vi "GV_CursorView.vi"(6 "pict in":picture, 8 "error in (no error)":errorcluster, 10 "Pos":cluster{"x":i16, "y":i16}, 11 "Gviewer in":refnum<class "Gviewer.lvclass">) -> (0 "error out":errorcluster, 3 "Gviewer out":refnum<class "Gviewer.lvclass">, 4 "pict out":picture)   [LabVIEW 2020, in "Sgraph_lib_V1.lvlib" / "Gviewer.lvclass"]
doc: "Andre Koelewijn, 11 aug 2021\n\nDraw cursor on canvas"
uses:
  Gviewer.lvclass
  Gviewer.lvclass/Gviewer.ctl
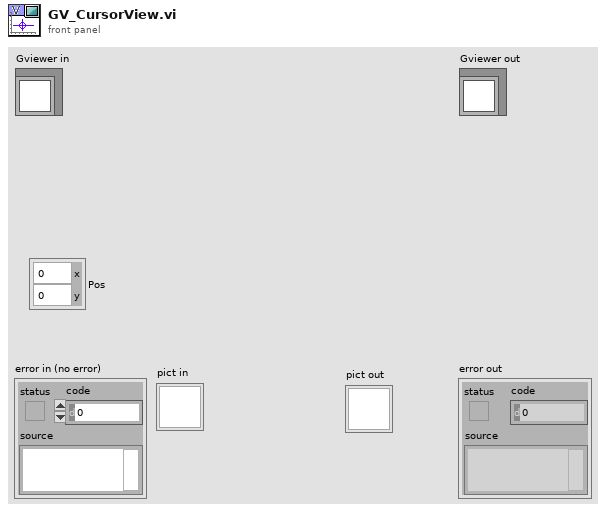
[diagram p1: front panel]
types:
  T1 = cluster{"Width":u16, "Style":enum32{"Solid", "Dash", "Dot", "DashDot", "DashDotDot"}}
  T2 = cluster{"horizontal":enum16{"left", "center", "right"}, "vertical":enum16{"top", "center", "bottom"}}
  T3 = typedef "Sgraph_lib_V1.lvlib/Gviewer.lvclass/Typedef_SelProperties.ctl" = cluster{"Color":u32, "LineType":T4, "max":dbl, "min":dbl, "unit":string}
  T4 = typedef "Sgraph_lib_V1.lvlib/Gviewer.lvclass/Typedef_LineType.ctl" = enum16{"num_bare", "num_MinMax_Area", "num_MinMax_Lines", "num_MinMax_Forfor", "num_Max_Area", "num_Max_Line", "num_Max_Forfor", "num_Min_Area", "num_Min_Line", "num_Min_Fosfor", "Boolean_Line_01", "Boolean_Area_01", "Boolean_Fosfor_01", "Boolean_Line_TF", "Boolean_Area_TF", "Boolean_Fosfor_TF", "Boolean_OnOff_Line", "Boolean_OnOff_Area", "Boolean_OnOff_Fosfor", "Boolean_spare", "StringEvent_Line", "StringEvent_TimeLine"}
  T5 = typedef "Sgraph_lib_V1.lvlib/DBAL.lvclass/DBAL_TAGprops.ctl" = T6[]
  T6 = typedef "Sgraph_lib_V1.lvlib/DBAL.lvclass/DBAL_TAGpropEdit.ctl" = cluster{"TAG":string, "Qtype":string, "TAGprop":T7}
  T7 = typedef "Sgraph_lib_V1.lvlib/typedef_com_TagProp.ctl" = cluster{"Description":string, "EngUnits":string, "RangeH":dbl, "RangeL":dbl, "Resolution":i32, "Obsolete":bool, "ChangeDate":timestamp, "ChangeSource":string, "ChangeReason":string, "TagFunc":u32}
  T8 = cluster{"data":dbl[], "max":dbl[], "min":dbl[], "Status":u32[]}[]
  T9 = cluster{"data":dbl[], "max":dbl[], "min":dbl[], "Status":u32[]}
  T10 = typedef "LVPositionTypeDef.ctl" = cluster{"Left":i32, "Top":i32}
  T11 = cluster{"left":i16, "top":i16, "right":i16, "bottom":i16}
  T12 = typedef "LVPoint32TypeDef.ctl" = cluster{"Horizontal":i32, "Vertical":i32}
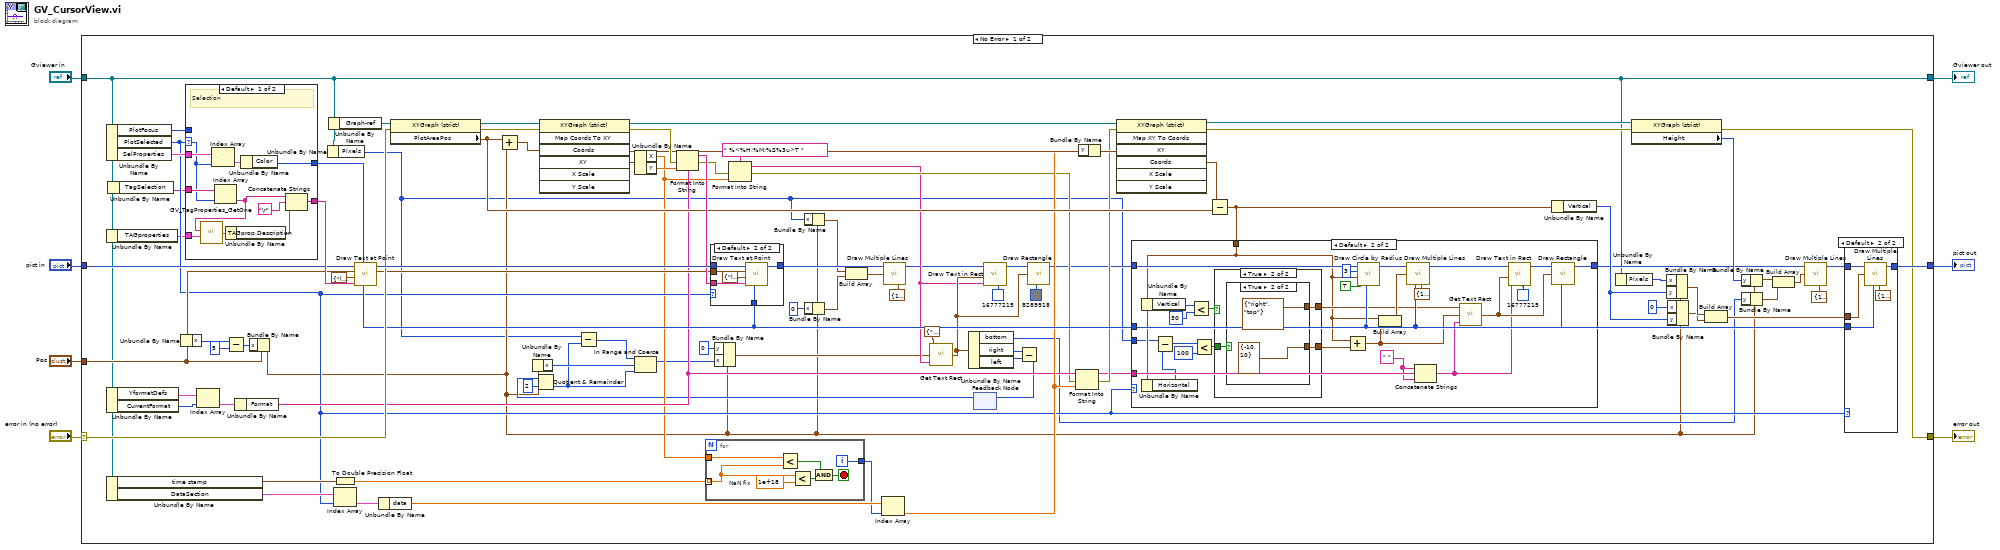
[diagram p0: block diagram]
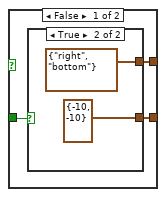
[diagram p3: hidden frame]
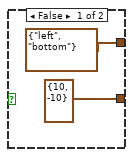
[diagram p4: hidden frame]
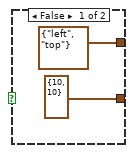
[diagram p5: hidden frame]
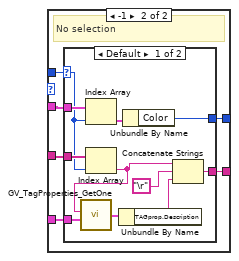
[diagram p8: hidden frame]
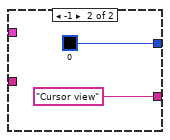
[diagram p9: hidden frame]
diagram:
  n1 = case shown="No Error" "error in (no error)" {
    selector: "error in (no error)" -> [w86 w193]
    tunnel: [w46 w193] -> w6
    tunnel: [w9 w192] -> w4
    tunnel: "Gviewer in" -> [w9 w192]
    tunnel: "pict in" -> [w89 w191]
    tunnel: [w49 w191] -> w2
    tunnel: "Pos" -> [w62 _]
    frame No Error {
      n2 = Unbundle By Name(w9) -> ("PlotFocus"=w52:i32, "PlotSelected"=w53:i32, "SelProperties"=w98:T3[])
      n3 = Unbundle By Name(w9) -> ("TAGproperties"=w8:T5)
      n4 = Unbundle By Name(w9) -> ("YformatDefs"=w81:cluster{"Description":string, "Format":string}[], "CurrentFormat"=w80:i32)
      n5 = Unbundle By Name(w9) -> ("time stamp"=w75:timestamp[], "DataSection"=w77:T8)
      n6 = Unbundle By Name(w9) -> ("TagSelection"=w10:string[])
      n7 = Unbundle By Name(w62) -> ("x"=w95:i16)
      n8 = case shown="Default" w53 {
        selector: w53 -> [w165 _]
        tunnel: w10 -> [w166 w174]
        tunnel: [w164 w177] -> w97
        tunnel: w98 -> [w169 w173]
        tunnel: [w170 w176] -> w59
        tunnel: w52 -> [_ w175]
        tunnel: w8 -> [w163 w172]
        frame Default {
          # "Selection"
          n9 = Index Array(array=w169, index=w165) -> (element=w171:T3)
          n10 = Index Array(array=w166, index=w165) -> (element=w162:string)
          n11 = call "GV_TagProperties_GetOne.vi"("TAG"=w162, "TAGproperties"=w163) -> ("TAGproperty"=w161:T6)  [unwired: 5 in]
          n12 = Unbundle By Name(w161) -> ("TAGprop.Description"=w168:string)
          n13 = Unbundle By Name(w171) -> ("Color"=w170:u32)
          n14 = Concatenate Strings(w162, "\r", w168) -> (w164:string)
        }
        frame -1 {
          # "No selection"
          n15 = case shown="Default" w175 {
            selector: w175 -> [w184 _]
            tunnel: [w181 "Cursor view"] -> w177
            tunnel: [w185 u32 0 ("Color")] -> w176
            tunnel: w174 -> [w188 _]
            tunnel: w173 -> [w187 _]
            tunnel: w172 -> [w180 _]
            frame Default {
              n16 = Index Array(array=w187, index=w184) -> (element=w186:T3)
              n17 = Index Array(array=w188, index=w184) -> (element=w179:string)
              n18 = call "GV_TagProperties_GetOne.vi"("TAG"=w179, "TAGproperties"=w180) -> ("TAGproperty"=w178:T6)  [unwired: 5 in]
              n19 = Unbundle By Name(w178) -> ("TAGprop.Description"=w183:string)
              n20 = Unbundle By Name(w186) -> ("Color"=w185:u32)
              n21 = Concatenate Strings(w179, "\r", w183) -> (w181:string)
            }
            frame -1 {
            }
          }
        }
      }
      n22 = Index Array(array=w81, index=w80) -> (element=w79:cluster{"Description":string, "Format":string})
      n23 = Subtract(x=w95, y=i16 5) -> (x-y=w93:i16)
      n24 = Unbundle By Name(w79) -> ("Format"=w57:string)
      n25 = Bundle By Name(cluster=w62, "x"=w93) -> (w16:cluster{"x":i16, "y":i16})
      n26 = Unbundle By Name(w9) -> ("Pixels"=w11:i32)
      n27 = Unbundle By Name(w9) -> ("Graph-ref"=w88:refnum<vi>)
      n28 = To Double Precision Float(number=w75) -> (double precision float=w74:dbl[])
      n29 = Index Array(array=w77, index=w53) -> (element=w76:T9)
      n30 = call <vilib>:"Draw Text at Point.vi"("text color(black)"=w59, "text"=w97, "alignment(left, top)"=T2 {"horizontal"=enum."left", "vertical"=enum."top"}, "origin"=w62, "picture"=w89) -> ("new picture"=w92:picture)  [unwired: 5 in, 1 out]
      n31 = Unbundle By Name(w76) -> ("data"=w73:dbl[])
      n32 = property class="XYGraph (strict)"(reference=w88, error in=w86) -> (reference out=w84:refnum<vi>, error out=w85:errorcluster, "PlotAreaPos"=w60:T10)
      n33 = Add(x=w60, y=w16) -> (x+y=w87:T10)
      n34 = Unbundle By Name(w16) -> ("x"=w35:i16)
      n35 = invoke class="XYGraph (strict)" method="Map Coords To XY"(reference=w84, error in=w85, "Coords"=w87) -> (reference out=w71:refnum<vi>, error out=w78:errorcluster, "XY"=w69:cluster{"X":dbl, "Y":dbl})  [unwired: 4 in, 4 out]
      n36 = Unbundle By Name(w69) -> ("X"=w50:dbl, "Y"=w83:dbl)
      n37 = Format Into String(format string=w57, error in=w78, w83) -> (resulting string=w82:string, error out=w48:errorcluster)  [unwired: 1 in]
      n38 = for {
        tunnel: w74 -> [w151] mode=indexing
        tunnel: w50 -> [w153]
        tunnel: [w152] -> w72
        i -> [w152]
        stop <- w147 stop-if-true
        w150 = 1e+18  # NaN fix
        n39 = Less?(x=w153, y=w151) -> (x < y?=w148:bool)
        n40 = Less?(x=w151, y=w150) -> (x < y?=w149:bool)
        n41 = And(x=w148, y=w149) -> (x .and. y?=w147:bool)
      }
      n42 = case shown="Default" w53 {
        tunnel: w92 -> [w154 w159]
        tunnel: [w154 w158] -> w25
        tunnel: w62 -> [_ w155]
        tunnel: w82 -> [_ w157]
        tunnel: w59 -> [_ w156]
        frame -1 {
        }
        frame Default {
          n43 = call <vilib>:"Draw Text at Point.vi"("text color(black)"=w156, "text"=w157, "alignment(left, top)"=T2 {"horizontal"=enum."left", "vertical"=enum."bottom"}, "origin"=w155, "picture"=w159) -> ("new picture"=w158:picture)  [unwired: 5 in, 1 out]
        }
      }
      n44 = Format Into String(format string=" %<%H:%M:%S%3u>T ", error in=w48, w50) -> (resulting string=w38:string, error out=w47:errorcluster)  [unwired: 1 in]
      n45 = Bundle By Name(cluster=w16, "x"=w11) -> (w21:cluster{"x":i16, "y":i16})
      n46 = Bundle By Name(cluster=w16, "x"=i16 0) -> (w22:cluster{"x":i16, "y":i16})
      n47 = Build Array(w21, w22) -> (w20:cluster{"x":i16, "y":i16}[])
      n48 = Index Array(array=w73, index=w72) -> (element=w58:dbl)
      n49 = call <vilib>:"Draw Multiple Lines.vi"("picture"=w25, "line endpoints"=w20, "pen"=T1 {"Width"=1, "Style"=enum."Dot"}) -> ("new picture"=w24:picture)  [unwired: 6 in]
      n50 = feedback #1() -> (w28:i16)  [unwired: 1 in]
      n51 = Quotient & Remainder(x=w28, y=i16 2) -> (floor(x/y)=w32:i16)  [unwired: 1 out]
      n52 = Subtract(x=w11, y=w32) -> (x-y=w33:i32)
      n53 = In Range and Coerce(upper limit=w33, x=w35, lower limit=w32) -> (coerced(x)=w34:i32)  [unwired: 1 out]
      n54 = Bundle By Name(cluster=w16, "y"=i16 0, "x"=w34) -> (w30:cluster{"x":i16, "y":i16})
      n55 = call <vilib>:"Get Text Rect.vi"("alignment(left, top)"=T2 {"horizontal"=enum."center", "vertical"=enum."top"}, "origin(0,0)"=w30, "text"=w38) -> ("rect"=w44:T11)  [unwired: 6 in]
      n56 = Unbundle By Name(w44) -> ("bottom"=w17:i16, "right"=w43:i16, "left"=w42:i16)
      n57 = call <vilib>:"Draw Text in Rect.vi"("BG color(transparent)"=u32 16777215, "text"=w38, "rect"=w44, "picture"=w24) -> ("new picture"=w45:picture)  [unwired: 7 in]
      n58 = Subtract(x=w43, y=w42) -> (x-y=w36:i16)
      n59 = feedback-in #1(w36) -> ()
      n60 = call <vilib>:"Draw Rectangle.vi"("picture"=w45, "rect"=w44, "color(black)"=u32 8289918 ("BG color(transparent)")) -> ("new picture"=w39:picture)  [unwired: 6 in]
      n61 = Format Into String(format string=w57, error in=w47, w58) -> (resulting string=w55:string, error out=w56:errorcluster)  [unwired: 1 in]
      n62 = Bundle By Name(cluster=w69, "Y"=w58) -> (w68:cluster{"X":dbl, "Y":dbl})
      n63 = invoke class="XYGraph (strict)" method="Map XY To Coords"(reference=w71, error in=w56, "XY"=w68) -> (reference out=w26:refnum<vi>, error out=w70:errorcluster, "Coords"=w63:T12)  [unwired: 4 in, 4 out]
      n64 = Subtract(x=w63, y=w60) -> (x-y=w54:T12)
      n65 = case shown="Default" w53 {
        tunnel: w39 -> [w99 w123]
        tunnel: [w99 w117] -> w18
        tunnel: w59 -> [_ w115]
        tunnel: w55 -> [_ w112]
        tunnel: w54 -> [_ w105]
        tunnel: w11 -> [_ w104]
        frame -1 {
        }
        frame Default {
          w110 = " "
          n66 = Unbundle By Name(w105) -> ("Vertical"=w109:i32)
          n67 = Unbundle By Name(w105) -> ("Horizontal"=w103:i32)
          n68 = Subtract(x=w104, y=w103) -> (x-y=w102:i32)
          n69 = Less?(x=w109, y=30) -> (x < y?=w107:bool)
          n70 = Less?(x=w102, y=100) -> (x < y?=w100:bool)
          n71 = case shown="True" w107 {
            tunnel: [w128 w135] -> w125
            tunnel: [w129 w136] -> w106
            tunnel: w100 -> [w127 w134]
            frame False {
              n72 = case shown="True" w127 {
                tunnel: [T2 {"horizontal"=enum."left", "vertical"=enum."bottom"} ("alignment(left, top)") T2 {"horizontal"=enum."right", "vertical"=enum."bottom"} ("alignment(left, top)")] -> w129
                tunnel: [cluster{"x":i16, "y":i16} {"x"=10, "y"=-10} ("ValuePosition") cluster{"x":i16, "y":i16} {"x"=-10, "y"=-10} ("ValuePosition")] -> w128
                frame False {
                }
                frame True {
                }
              }
            }
            frame True {
              n73 = case shown="True" w134 {
                tunnel: [T2 {"horizontal"=enum."left", "vertical"=enum."top"} ("alignment(left, top)") T2 {"horizontal"=enum."right", "vertical"=enum."top"} ("alignment(left, top)")] -> w136
                tunnel: [cluster{"x":i16, "y":i16} {"x"=10, "y"=10} ("ValuePosition") cluster{"x":i16, "y":i16} {"x"=-10, "y"=10} ("ValuePosition")] -> w135
                frame False {
                }
                frame True {
                }
              }
            }
          }
          n74 = Add(x=w105, y=w125) -> (x+y=w113:T12)
          n75 = call <vilib>:"Draw Circle by Radius.vi"("color(black)"=w115, "fill?(F)"=TRUE, "pixel center"=w105, "radius"=i16 3, "picture"=w123) -> ("new picture"=w121:picture)  [unwired: 6 in]
          n76 = Build Array(w105, w113) -> (w120:T12[])
          n77 = call <vilib>:"Draw Multiple Lines.vi"("picture"=w121, "line endpoints"=w120, "color(black)"=w115, "pen"=T1 {"Width"=1, "Style"=enum."Solid"}) -> ("new picture"=w119:picture)  [unwired: 5 in]
          n78 = Concatenate Strings(w110, w112, w110) -> (w111:string)
          n79 = call <vilib>:"Get Text Rect.vi"("alignment(left, top)"=w106, "origin(0,0)"=w113, "text"=w111) -> ("rect"=w116:T11)  [unwired: 6 in]
          n80 = call <vilib>:"Draw Text in Rect.vi"("BG color(transparent)"=u32 16777215, "text"=w111, "rect"=w116, "picture"=w119) -> ("new picture"=w118:picture)  [unwired: 7 in]
          n81 = call <vilib>:"Draw Rectangle.vi"("picture"=w118, "rect"=w116, "color(black)"=w115) -> ("new picture"=w117:picture)  [unwired: 6 in]
        }
      }
      n82 = Unbundle By Name(w54) -> ("Vertical"=w61:i32)
      n83 = Unbundle By Name(w9) -> ("Pixels"=w15:i32)
      n84 = property class="XYGraph (strict)"(reference=w26, error in=w70) -> (error out=w46:errorcluster, "Height"=w27:u32)  [unwired: 1 out]
      n85 = Bundle By Name(cluster=w16, "x"=w15, "y"=w61) -> (w65:cluster{"x":i16, "y":i16})
      n86 = Bundle By Name(cluster=w16, "x"=i16 0, "y"=w61) -> (w64:cluster{"x":i16, "y":i16})
      n87 = Build Array(w65, w64) -> (w66:cluster{"x":i16, "y":i16}[])
      n88 = Bundle By Name(cluster=w16, "y"=w27) -> (w14:cluster{"x":i16, "y":i16})
      n89 = Bundle By Name(cluster=w16, "y"=w17) -> (w13:cluster{"x":i16, "y":i16})
      n90 = Build Array(w14, w13) -> (w90:cluster{"x":i16, "y":i16}[])
      n91 = call <vilib>:"Draw Multiple Lines.vi"("picture"=w18, "line endpoints"=w90, "pen"=T1 {"Width"=1, "Style"=enum."Dot"}) -> ("new picture"=w67:picture)  [unwired: 6 in]
      n92 = case shown="Default" w53 {
        tunnel: w67 -> [w141 w145]
        tunnel: [w141 w144] -> w49
        tunnel: w66 -> [_ w143]
        tunnel: w59 -> [_ w142]
        frame -1 {
        }
        frame Default {
          n93 = call <vilib>:"Draw Multiple Lines.vi"("picture"=w145, "line endpoints"=w143, "color(black)"=w142, "pen"=T1 {"Width"=1, "Style"=enum."Dot"}) -> ("new picture"=w144:picture)  [unwired: 5 in]
        }
      }
    }
    frame Error {
    }
  }
  "error out" <- w6
  "Gviewer out" <- w4
  "pict out" <- w2
